vi "Destroy Error Pointer.vi"(8 "error in (no error)":errorcluster, 11 "Thread in":refnum<class "Thread.lvclass">) -> (0 "error out":errorcluster, 3 "Thread out":refnum<class "Thread.lvclass">)   [LabVIEW 2019, in "DSF Core.lvlib" / "Thread.lvclass"]
uses:
  Thread.lvclass
  Thread.lvclass/Thread.ctl
  Pointers/Error/Error Pointer.lvclass
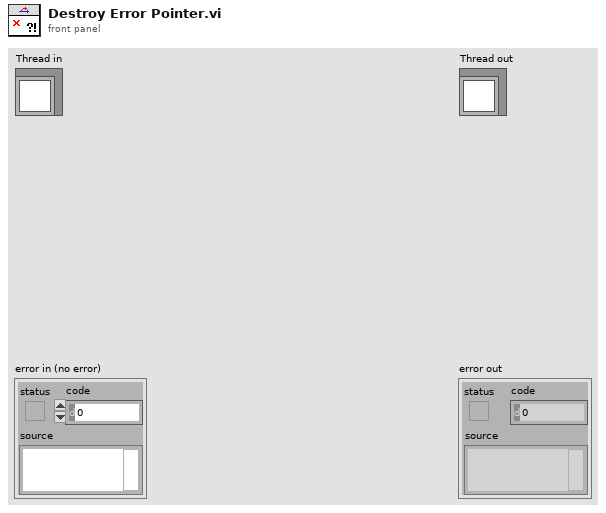
[diagram p1: front panel]
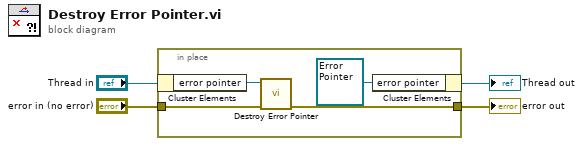
[diagram p0: block diagram]
diagram:
  n1 = in-place {
    in-place-border: [w7] -> w3
    in-place-border: "error in (no error)" -> [w8]
    n2 = in-place-cluster #1("Thread in") -> ("error pointer"=w6:refnum<class "Error Pointer.lvclass">)
    n3 = call "Destroy Error Pointer.vi"("error in (no error)"=w8, "Error Pointer in"=w6) -> ("error out"=w7:errorcluster)  [unwired: 9 in]
    n4 = in-place-cluster #1("error pointer"=refnum<class "Error Pointer.lvclass"> refnum) -> (→"Thread out":refnum<class "Thread.lvclass">)
  }
  "error out" <- w3
